vi "ROI entry- populate lbox headers.vi"(8 "error in (no error)":errorcluster) -> (0 "error out":errorcluster)   [LabVIEW 2020]
uses:
  Visualisation/Functional Imaging Viewer/Typedefs/ROI parameters data type.ctl
  Globals/gl_ROI Entry UI globals.vi
panel:
  out "Names":string[](array[string])
  in  "X-Y-Z coordinates":T1 {"Apparent Frame Size" format="%#_6f"; "Original FOV (um)" format="%#_6f"; "Pixels per miniscan" format="%#_6f"; "Dwell Time per pixel" format="%#_6f"; "Resolution" format="%#_6f"; "ROI group ID" format="%#_6f"; "Laser Power (%)" format="%#_6f"; "Zoom" format="%#_6f"; "Frame Size" format="%#_6f"; "Number of lines" format="%#_6f"; "Composite ID" format="%#_6f"; "Angle (deg)" format="%#_6f"; "ROI Time (ns)" format="%#_6f"; "ROI ID" format="%#_6f"; "Pixels in ROI" format="%#_6f"; "ROI index" format="%#_6f"; "Z stop" format="%#_6f"; "Y stop" format="%#_6f"; "X stop" format="%#_6f"; "Z start" format="%#_6f"; "X start" format="%#_6f"; "Y start" format="%#_6f"}
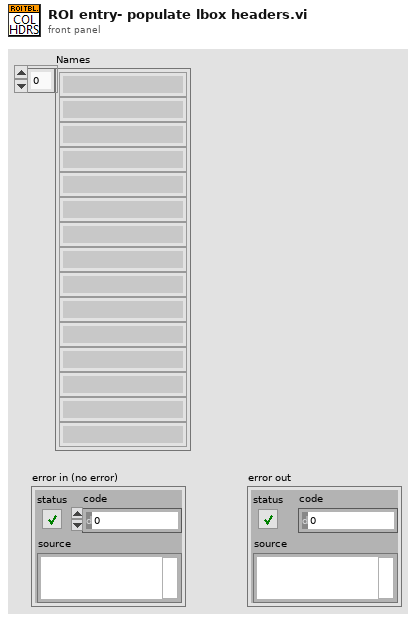
[diagram p1: front panel]
types:
  T1 = typedef "ROI parameters data type.ctl" = cluster{"ROI index":dbl, "ROI ID":dbl, "ROI Time (ns)":dbl, "Pixels in ROI":dbl, "X start":dbl, "Y start":dbl, "Z start":dbl, "X stop":dbl, "Y stop":dbl, "Z stop":dbl, "Angle (deg)":dbl, "Composite ID":dbl, "Number of lines":dbl, "Frame Size":dbl, "Zoom":dbl, "Laser Power (%)":dbl, "ROI group ID":dbl, "Resolution":dbl, "Dwell Time per pixel":dbl, "Pixels per miniscan":dbl, "Original FOV (um)":dbl, "Apparent Frame Size":dbl, "Z Plane Idx":i32[], "Z Plane codes":i32[]}
  T2 = typedef "ROI entry screen ctrl refs cluster.ctl" = cluster{"Done button":refnum<vi>, "Imaging button":refnum<vi>, "Acquisition button":refnum<vi>, "Scan dwell time per pixel (us)":refnum<vi>, "# of planes":refnum<vi>, "Zoom Ctrl":refnum<vi>, "Equal size":refnum<vi>, "Channel":refnum<vi>, "Image Display":refnum<vi>, "Z-Plane Selector":refnum<vi>, "Number of lines left":refnum<vi>, "Z-stack folder path":refnum<vi>, "POI Density":refnum<vi>, "Arb Plane Entry":refnum<vi>, "Whole Plane":refnum<vi>, "Line Mode":refnum<vi>, "Clear Last":refnum<vi>, "Clear All":refnum<vi>, "Delete Lines":refnum<vi>, "Trial Length (sec)":refnum<vi>, "Palette Type":refnum<vi>, "Intensity slider":refnum<vi>, "# POI":refnum<vi>, "Max Z Proj":refnum<vi>, "Zplane ind":refnum<vi>, "Wavelength (nm)":refnum<vi>, "Number of Trials":refnum<vi>, "Funct stim.trig.enable":refnum<vi>, "Funct stim.trig.delay (s)":refnum<vi>, "Line Mode":refnum<vi>, "Step size (µm)":refnum<vi>, "ROI move mode":refnum<vi>, "Cool-down time (s)":refnum<vi>, "Enable cool-down time":refnum<vi>, "Motor Z ind. (um)":refnum<vi>, "AOL Z ind. (um)":refnum<vi>, "Load Reference Image":refnum<vi>, "Rel.  Res.":refnum<vi>, "ROI LIST":refnum<vi>, "Show All":refnum<vi>, "ROI Type":refnum<vi>, "Start Plane":refnum<vi>, "Stop Plane":refnum<vi>, "Offset ROI":refnum<vi>, "Tab Control":refnum<vi>, "Laser Power(%)":refnum<vi>, "Cycle rate":refnum<vi>, "FOV (Ind.)":refnum<vi>, "Frame Size (Ind.)":refnum<vi>, "Resolution (Ind.)":refnum<vi>, "Pixel Density (Ind)":refnum<vi>, "Laser Power (Ind.)":refnum<vi>, "Dwell Time (Ind.)":refnum<vi>, "Adj MC":refnum<vi>}
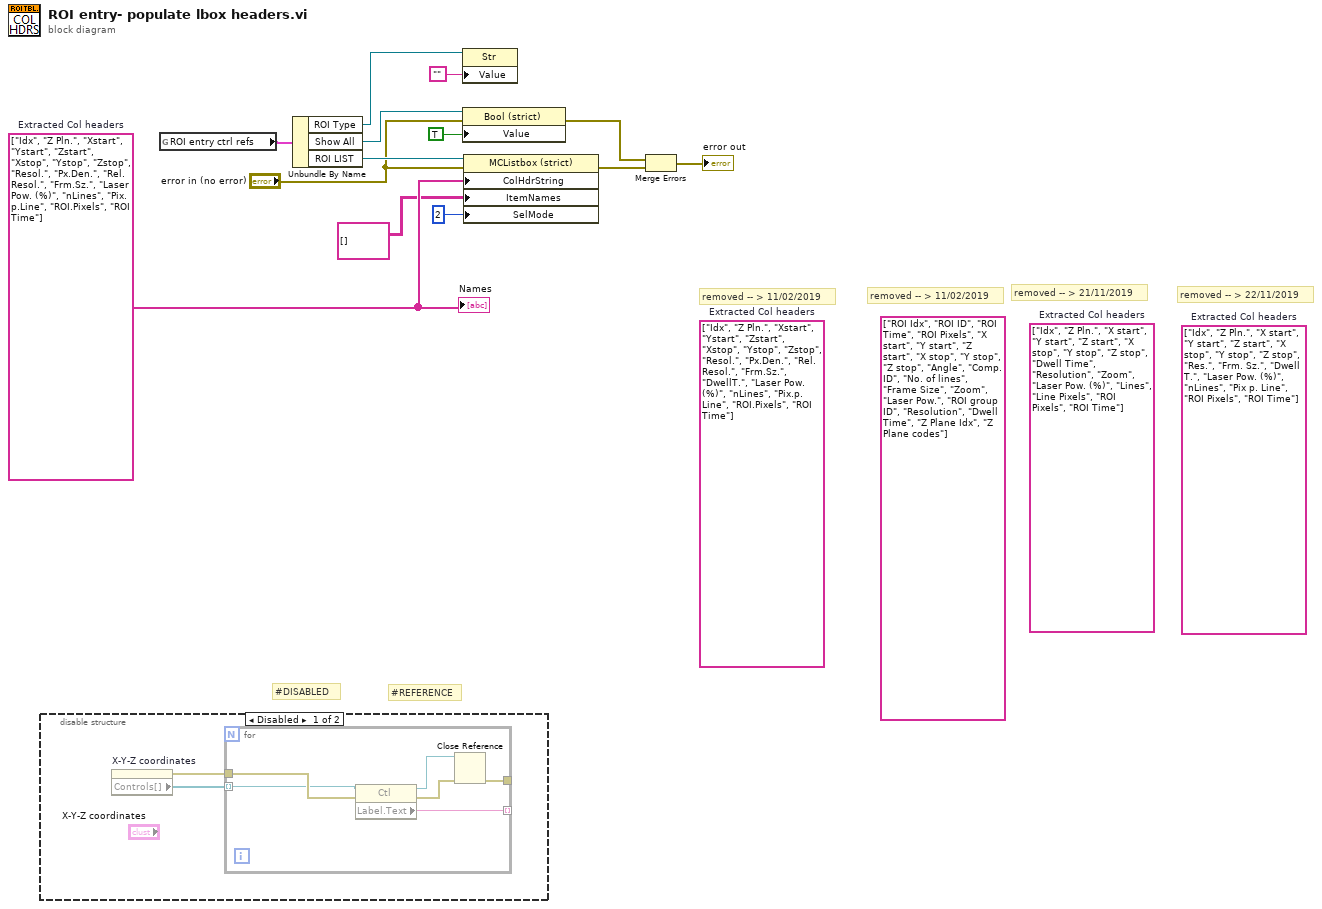
[diagram p0: block diagram]
diagram:
  (unwired) string[] ["Idx", "Z Pln.", "Xstart", "Ystart", "Zstart", "Xstop", "Ystop", "Zstop", "Resol.", "Px.Den.", "Rel.Resol.", "Frm.Sz.", "DwellT.", "Laser Pow. (%)", "nLines", "Pix.p.Line", "ROI.Pixels", "ROI Time"]  # Extracted Col headers
  (unwired) string[] ["Idx", "Z Pln.", "X start", "Y start", "Z start", "X stop", "Y stop", "Z stop", "Res.", "Frm. Sz.", "Dwell T.", "Laser Pow. (%)", "nLines", "Pix p. Line", "ROI Pixels", "ROI Time"]  # Extracted Col headers
  (unwired) string[] ["Idx", "Z Pln.", "X start", "Y start", "Z start", "X stop", "Y stop", "Z stop", "Dwell Time", "Resolution", "Zoom", "Laser Pow. (%)", "Lines", "Line Pixels", "ROI Pixels", "ROI Time"]  # Extracted Col headers
  w11 = string[] ["Idx", "Z Pln.", "Xstart", "Ystart", "Zstart", "Xstop", "Ystop", "Zstop", "Resol.", "Px.Den.", "Rel.Resol.", "Frm.Sz.", "Laser Pow. (%)", "nLines", "Pix.p.Line", "ROI.Pixels", "ROI Time"]  # Extracted Col headers
  (unwired) string[] ["ROI Idx", "ROI ID", "ROI Time", "ROI Pixels", "X start", "Y start", "Z start", "X stop", "Y stop", "Z stop", "Angle", "Comp. ID", "No. of lines", "Frame Size", "Zoom", "Laser Pow.", "ROI group ID", "Resolution", "Dwell Time", "Z Plane Idx", "Z Plane codes"] ("Array 2")
  # "removed -- > 11/02/2019"
  # "removed -- > 11/02/2019"
  # "removed -- > 22/11/2019"
  # "removed -- > 21/11/2019"
  # "#REFERENCE"
  # "#DISABLED"
  n1 = disable-structure shown="Disabled" {
    frame Disabled {
      n2 = property on="X-Y-Z coordinates" class="Clust (strict)"() -> (error out=w15:errorcluster, "Controls[]"=w14:refnum<vi>[])  [unwired: 2 in, 1 out]
      n3 = for {
        tunnel: w15 -> [w21]
        tunnel: w14 -> [w20] mode=indexing
        tunnel: [w19] -> _ mode=indexing
        tunnel: [w16] -> _
        n4 = property class="Ctl"(reference=w20, error in=w21) -> (reference out=w17:refnum<vi>, error out=w18:errorcluster, "Label.Text"=w19:string)
        n5 = Close Reference(reference=w17, error in (no error)=w18) -> (error out=w16:errorcluster)
      }
    }
    frame Enabled {
    }
  }
  n6 = global read "gl_ROI Entry UI globals.vi" "ROI entry ctrl refs"() -> (w12:T2)
  n7 = Unbundle By Name(w12) -> ("ROI Type"=w2:refnum<vi>, "Show All"=w5:refnum<vi>, "ROI LIST"=w13:refnum<vi>)
  n8 = property class="Str"(reference=w2, "Value"="") -> ()  [unwired: 1 in, 2 out]
  n9 = property class="Bool (strict)"(reference=w5, error in="error in (no error)", "Value"=TRUE) -> (error out=w7:errorcluster)  [unwired: 1 out]
  n10 = property class="MCListbox (strict)"(reference=w13, error in="error in (no error)", "ColHdrString"=w11, "ItemNames"=string[][] [], "SelMode"=2 ("Selection Mode")) -> (error out=w6:errorcluster)  [unwired: 1 out]
  n11 = Merge Errors(w7, w6) -> (→"error out":errorcluster)
  "Names" <- w11
